vi "RT_StartStopStreaming.vi"(8 "error in (no error)":errorcluster, 11 "Start/Stop?":bool) -> (0 "error out":errorcluster)   [LabVIEW 2020]
uses:
  <vilib>/FPGAPlugInAG/cRIO-9040/niLvFpga_Open_cRIO-9040.vi
  <vilib>/Utility/error.llb/Error Cluster From Error Code.vi
  <vilib>/rvi/errors/niLvFpgaAdjustHostInterfaceError.vi
  <vilib>/rvi/interface/nirviOpenFPGA/nirviOpenFPGA.xnode
  FPGA Bitfiles/depapp_FPGATarget_FPGAmain_WC8wSYHNwdY.lvbitx
  FPGA_main.vi
  <vilib>/rvi/interface/nirviReadWriteControl/nirviReadWriteControl.xnode
  NiFpgaLv.dll
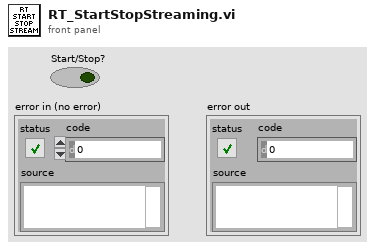
[diagram p1: front panel]
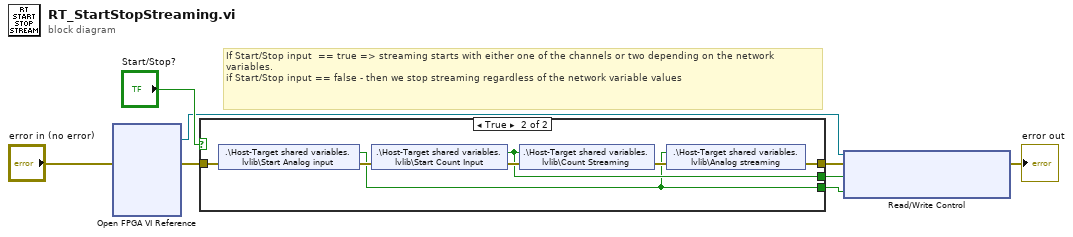
[diagram p0: block diagram]
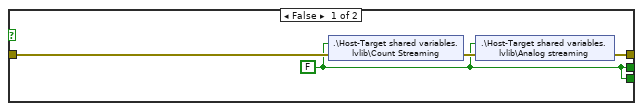
[diagram p2: hidden frame]
diagram:
  # "If Start/Stop input  == true => streaming starts with either one of the channels or two depending on the network \nvariables. \nif Start/Stop input == false - then we stop streaming regardless of the network variable values"
  n1 = xnode "Open FPGA VI Reference"("error in"="error in (no error)") -> ("FPGA VI Reference Out"=w5:refnum<k20>, "error out"=w6:errorcluster)  [unwired: 1 in]
  n2 = case shown="True" "Start/Stop?" {
    tunnel: w6 -> [w12 w16]
    tunnel: [w10 w15] -> w4
    tunnel: [w9 w14] -> w3
    tunnel: [w9 w13] -> w2
    frame False {
      w9 = FALSE ("Boolean")
      n3 = shared-variable ".\\Host-Target shared variables.lvlib\\Count Streaming"(w9, error in=w12) -> (error out=w11:errorcluster)
      n4 = shared-variable ".\\Host-Target shared variables.lvlib\\Analog streaming"(w9, error in=w11) -> (error out=w10:errorcluster)
    }
    frame True {
      n5 = shared-variable ".\\Host-Target shared variables.lvlib\\Start Analog input"(error in=w16) -> (w13:bool, error out=w17:errorcluster)
      n6 = shared-variable ".\\Host-Target shared variables.lvlib\\Start Count Input"(error in=w17) -> (w14:bool, error out=w18:errorcluster)
      n7 = shared-variable ".\\Host-Target shared variables.lvlib\\Count Streaming"(w14, error in=w18) -> (error out=w19:errorcluster)
      n8 = shared-variable ".\\Host-Target shared variables.lvlib\\Analog streaming"(w13, error in=w19) -> (error out=w15:errorcluster)
    }
  }
  n9 = xnode "Read/Write Control"("FPGA VI Reference In"=w5, "error in"=w4, "Stream counts?"=w3, "Stream  AI"=w2) -> ("error out"=→"error out":errorcluster)  [unwired: 1 out]
